vi "Gui_Fill_List_From_File.vi"(8 "error in (no error)":errorcluster, 9 "Resource Name":string="Users.txt", 10 "Resource Path":path=path "D:/S.O.F.T.S/LABVIEW/PIL/resources", 11 "Refnum LstDér":refnum<vi>) -> (0 "error out":errorcluster, 2 "Table":string[](array[string]), 3 "Refnum LstDér out":refnum<vi>)   [LabVIEW 2018]
panel:
  in  "List":i32[](listbox)
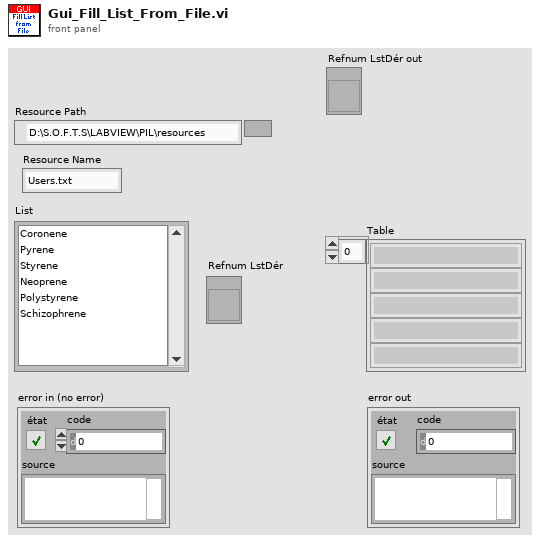
[diagram p1: front panel]
types:
  T1 = enum16{"open", "replace", "create", "open or create", "replace or create", "replace or create with confirmation"}
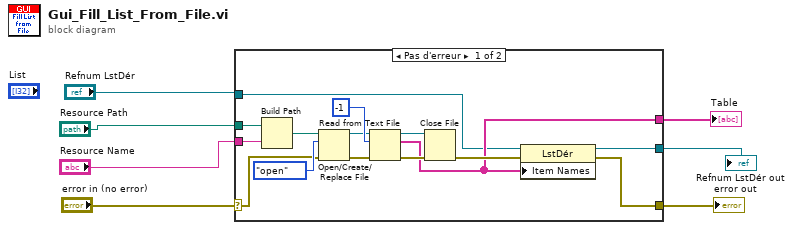
[diagram p0: block diagram]
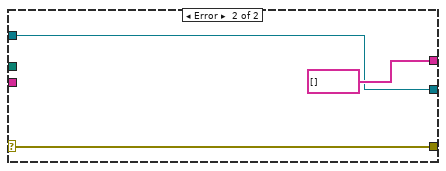
[diagram p2: hidden frame]
diagram:
  n1 = case shown="Pas d'erreur" "error in (no error)" {
    selector: "error in (no error)" -> [w10 w25]
    tunnel: "Resource Path" -> [w22 _]
    tunnel: "Resource Name" -> [w21 _]
    tunnel: [w12 string[] []] -> w3
    tunnel: [w9 w25] -> w4
    tunnel: "Refnum LstDér" -> [w11 w23]
    tunnel: [w8 w23] -> w1
    frame No Error {
      n2 = Build Path(base path=w22, name or relative path=w21) -> (appended path=w18:path)
      n3 = Open/Create/Replace File ("Ouvrir/Créer/Remplacer un fichier")(file path (use dialog)=w18, error in=w10, operation (0:open)=T1."open") -> (refnum out=w19:refnum<file>, error out=w16:errorcluster)  [unwired: 3 in, 1 out]
      n4 = Read from Text File ("Lire un fichier texte")(file (use dialog)=w19, count=-1 ("nombre"), error in=w16) -> (refnum out=w14:refnum<file>, text=w12:string[], error out=w15:errorcluster)  [unwired: 1 in, 1 out]
      n5 = Close File(refnum=w14, error in=w15) -> (error out=w13:errorcluster)  [unwired: 1 out]
      n6 = property class="LstDér"(reference=w11, error in=w13, "Item Names"=w12) -> (reference out=w8:refnum<vi>, error out=w9:errorcluster)
    }
    frame Error {
    }
  }
  "Table" <- w3
  "error out" <- w4
  "Refnum LstDér out" <- w1
